vi "TF_MotorCurrentInput.vi"(1 "Motor Current Monitor Value [V]":dbl) -> (0 "Current [A]":dbl)   [LabVIEW 2019]
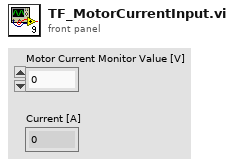
[diagram p1: front panel]
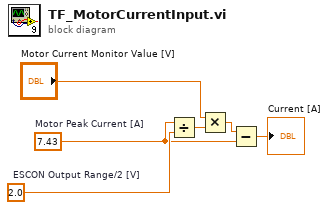
[diagram p0: block diagram]
diagram:
  w5 = 2.0  # ESCON Output Range/2 [V]
  w3 = 7.43  # Motor Peak Current [A]
  n1 = Divide(x=w3, y=w5) -> (x/y=w2:dbl)
  n2 = Multiply(x="Motor Current Monitor Value [V]", y=w2) -> (x*y=w1:dbl)
  n3 = Subtract(x=w1, y=w3) -> (x-y=→"Current [A]":dbl)
